vi "Get Raw Set.vi"(0 "DBSet in":refnum<class "DBSet.lvclass">, 11 "error in (no error)":errorcluster {"code" format="Error %.0f"}) -> (4 "DBSet out":refnum<class "DBSet.lvclass">, 6 "Raw Set":string[](array[string]), 15 "error out":errorcluster {"code" format="Error %.0f"})   [LabVIEW 2020, in "DBSet.lvclass"]
uses:
  DBSet.lvclass
  DBSet.lvclass/DBSet.ctl
  <vilib>/drjdpowell/SQLite Library/SQLite.lvlib
  <vilib>/drjdpowell/SQLite Library/SQL Connection/Execute SQL (1D String).vi
  <vilib>/drjdpowell/SQLite Library/SQL Connection/Connection.lvclass
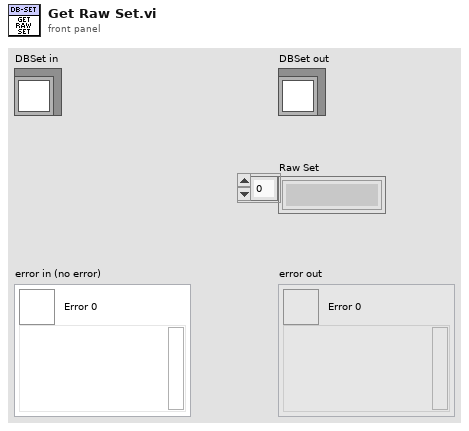
[diagram p1: front panel]
types:
  T1 = typedef "Semaphore RefNum" = refnum<k1>
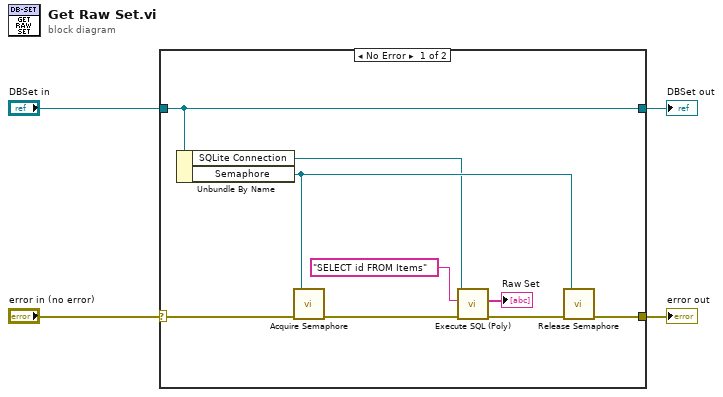
[diagram p0: block diagram]
diagram:
  n1 = case shown="No Error" "error in (no error)" {
    selector: "error in (no error)" -> [w12 w15]
    tunnel: [w11 w15] -> w3
    tunnel: [w13 w14] -> w1
    tunnel: "DBSet in" -> [w13 w14]
    frame No Error {
      n2 = Unbundle By Name(w13) -> ("SQLite Connection"=w7:refnum<class "Connection.lvclass">, "Semaphore"=w10:T1)
      n3 = call <vilib>:"Acquire Semaphore.vi"("error in (no error)"=w12, "semaphore"=w10) -> ("error out"=w9:errorcluster)  [unwired: 3 in, 2 out]
      n4 = call-poly <vilib>:"Execute SQL (Poly).vi"("error in (no error)"=w9, "SQL"="SELECT id FROM Items", "SQLite Connection in"=w7) -> ("error out"=w8:errorcluster, "Result Set"=→"Raw Set":string[])  [unwired: 5 in, 2 out]
      n5 = call <vilib>:"Release Semaphore.vi"("error in (no error)"=w8, "semaphore"=w10) -> ("error out"=w11:errorcluster)  [unwired: 4 in, 1 out]
    }
    frame Error {
    }
  }
  "error out" <- w3
  "DBSet out" <- w1
